vi "test_DAC.vi"() -> ()   [LabVIEW 2019]
uses:
  <vilib>/DAQmx/write.llb/DAQmx Write (Analog Wfm 1Chan NSamp).vi
  <vilib>/DAQmx/create/channels.llb/DAQmx Create Channel (AO-Voltage-Basic).vi
  <vilib>/DAQmx/configure/timing.llb/DAQmx Timing (Use Waveform).vi
  <vilib>/DAQmx/miscellaneous.llb/DAQmx Fill In Error Info.vi
panel:
  out "message":string
  out "wf_graph":waveform(dbl)(graph)
  in  "waveform":T1(ring)
  in  "N_steps":i32=100
  in  "T_sweep":dbl=1.0
  in  "N_sweeps":i32=2
  in  "channel":tag="Dev1/ao0"
  # "s"
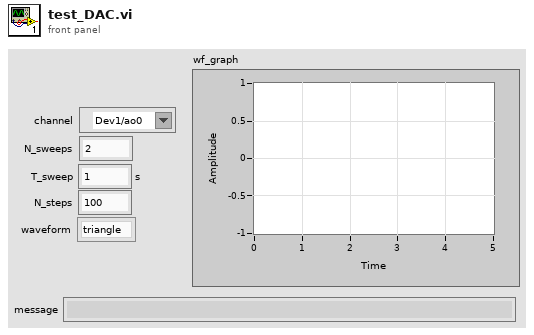
[diagram p1: front panel]
types:
  T1 = enum16{"triangle", "saw_direct", "saw_invert", "sine"}
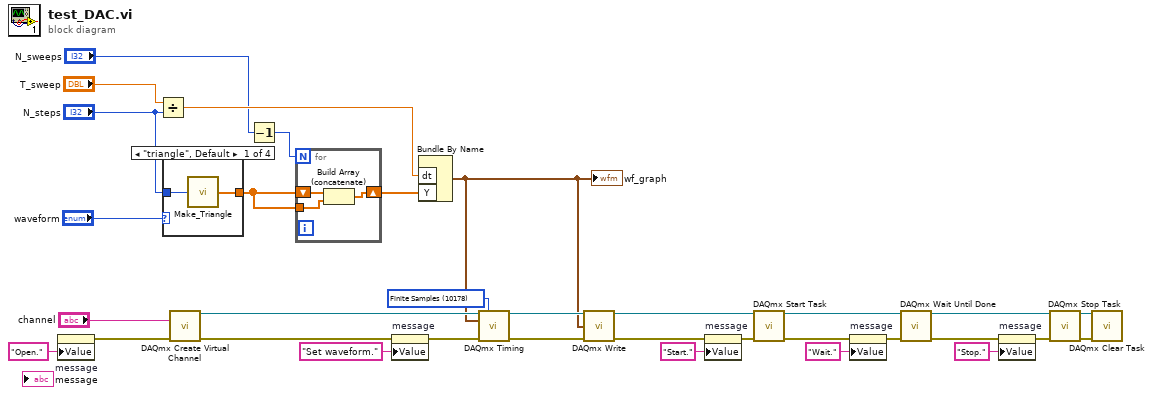
[diagram p0: block diagram]
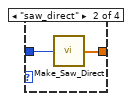
[diagram p2: hidden frame]
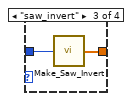
[diagram p3: hidden frame]
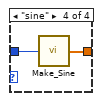
[diagram p4: hidden frame]
diagram:
  w32 = 10178 items=["Finite Samples"=10178, "Continuous Samples"=10123, "Hardware Timed Single Point"=12522] ("sample mode")
  n1 = property on="message" class="Str"("Value"="Open." ("message")) -> (error out=w14:errorcluster)  [unwired: 2 in, 1 out]
  n2 = Divide(x="T_sweep", y="N_steps") -> (x/y=w21:dbl)
  n3 = case shown="\"triangle\", Default" "waveform" {
    tunnel: "N_steps" -> [w35 w37 w39 w41]
    tunnel: [w34 w36 w38 w40] -> w22
    frame "triangle", Default {
      n4 = call "Make_Triangle.vi"("N_steps_1"=w35) -> ("TriangleWaveform"=w34:dbl[])
    }
    frame "saw_direct" {
      n5 = call "Make_Saw_Direct.vi"("N_steps_1"=w37) -> ("SawDirectWaveform"=w36:dbl[])
    }
    frame "saw_invert" {
      n6 = call "Make_Saw_Invert.vi"("N_steps_1"=w39) -> ("SawInvertWaveform"=w38:dbl[])
    }
    frame "sine" {
      n7 = call "Make_Sine.vi"("N_steps_1"=w41) -> ("SineWaveform"=w40:dbl[])
    }
  }
  n8 = call-poly <vilib>:"DAQmx Create Virtual Channel.vi"("physical channels"="channel", "error in"=w14) -> ("task out"=w24:refnum<k21>, "error out"=w12:errorcluster)  [unwired: 12 in]
  n9 = Decrement(x="N_sweeps") -> (x-1=w20:i32)
  n10 = for {
    N: w20 -> [_]
    shift-right: [w42] -> w23
    shift-left: w22 -> [w44]
    tunnel: w22 -> [w43]
    n11 = Build Array (concatenate)(w44, w43) -> (w42:dbl[])
  }
  n12 = property on="message" class="Str"(error in=w12, "Value"="Set waveform." ("message")) -> (error out=w11:errorcluster)  [unwired: 1 in, 1 out]
  n13 = Bundle By Name("dt"=w21, "Y"=w23) -> (w15:waveform(dbl))  [unwired: 1 in]
  "wf_graph" <- w15
  n14 = call-poly <vilib>:"DAQmx Timing.vi"("task/channels in"=w24, "sample mode"=w32, "waveform"=w15, "error in"=w11) -> ("task out"=w26:refnum<k21>, "error out"=w25:errorcluster)  [unwired: 10 in]
  n15 = call-poly <vilib>:"DAQmx Write.vi"("task/channels in"=w26, "data"=w15, "error in"=w25) -> ("task out"=w27:refnum<k21>, "error out"=w9:errorcluster)  [unwired: 10 in, 1 out]
  n16 = property on="message" class="Str"(error in=w9, "Value"="Start." ("message")) -> (error out=w8:errorcluster)  [unwired: 1 in, 1 out]
  n17 = call <vilib>:"DAQmx Start Task.vi"("task/channels in"=w27, "error in"=w8) -> ("task out"=w31:refnum<k21>, "error out"=w7:errorcluster)  [unwired: 12 in]
  n18 = property on="message" class="Str"(error in=w7, "Value"="Wait." ("message")) -> (error out=w6:errorcluster)  [unwired: 1 in, 1 out]
  n19 = call <vilib>:"DAQmx Wait Until Done.vi"("task/channels in"=w31, "error in"=w6) -> ("task out"=w30:refnum<k21>, "error out"=w5:errorcluster)  [unwired: 12 in]
  n20 = property on="message" class="Str"(error in=w5, "Value"="Stop." ("message")) -> (error out=w4:errorcluster)  [unwired: 1 in, 1 out]
  n21 = call <vilib>:"DAQmx Stop Task.vi"("task/channels in"=w30, "error in"=w4) -> ("task out"=w29:refnum<k21>, "error out"=w28:errorcluster)  [unwired: 12 in]
  n22 = call <vilib>:"DAQmx Clear Task.vi"("task in"=w29, "error in"=w28) -> ()  [unwired: 13 in, 1 out]
